vi "FindAnalogPulsePositions.vi"(9 "t0":dbl format="%#_13g", 10 "level":dbl format="%#_13g", 11 "tach signal":waveform(dbl)) -> (3 "pulse positions":dbl[](array[numeric]))   [LabVIEW 2017, in "CmsAcquisition.lvlib"]
uses:
  <vilib>/addons/InsightCM/Devices/Shared/Cms/CmsAcquisition/CmsAcquisition.lvlib
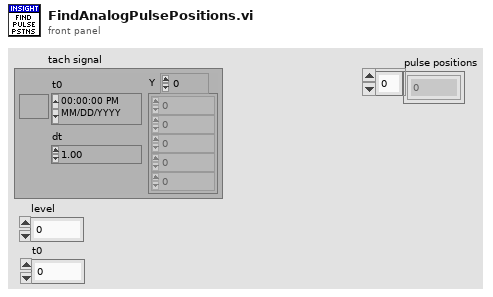
[diagram p1: front panel]
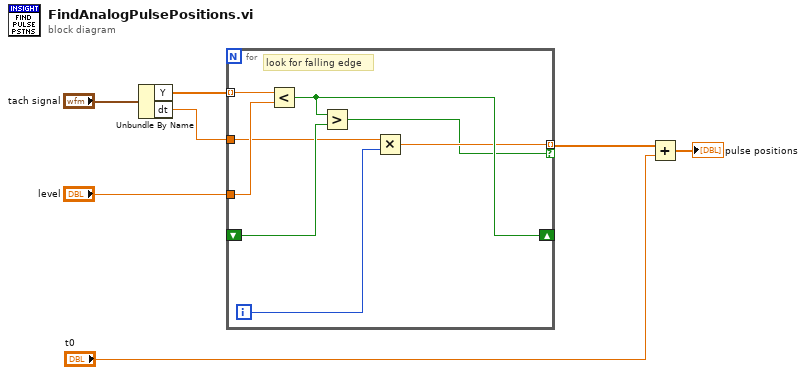
[diagram p0: block diagram]
diagram:
  n1 = Unbundle By Name("tach signal") -> ("Y"=w5:dbl[], "dt"=w4:dbl)
  n2 = for {
    tunnel: "level" -> [w14]
    tunnel: w5 -> [w15] mode=indexing
    shift-right: [w13] -> _
    shift-left: _ -> [w12]
    tunnel: w4 -> [w11]
    tunnel: [w9] -> w3 mode=indexing if=w8
    i -> [w10]
    # "look for falling edge"
    n3 = Less?(x=w15, y=w14) -> (x < y?=w13:bool)
    n4 = Greater?(x=w13, y=w12) -> (0:w8:bool)
    n5 = Multiply(x=w11, y=w10) -> (x*y=w9:dbl)
  }
  n6 = Add(x=w3, y="t0") -> (x+y=→"pulse positions":dbl[])
